vi "Read Data Type.vi"(8 "error in (no error)":errorcluster, 11 "Channel in":refnum<class "Channel.lvclass">) -> (0 "error out":errorcluster, 2 "Data Type":T1, 3 "Channel out":refnum<class "Channel.lvclass">)   [LabVIEW 2013, in "Channel.lvclass"]
uses:
  Channel.lvclass
  channel_dataType.ctl
  Channel.lvclass/Channel.ctl
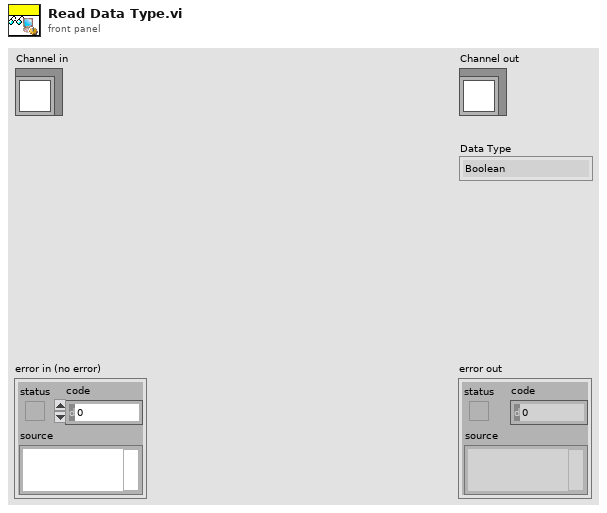
[diagram p1: front panel]
types:
  T1 = typedef "Channel.lvclass/channel_dataType.ctl" = enum16{"Boolean", "U8", "I8", "U16", "I16", "U32", "I32", "U64", "I64", "FXPI32", "FXPU32", "FXPI64", "FXPU64", "PWM"}
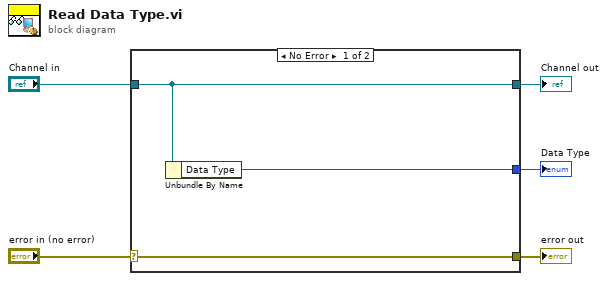
[diagram p0: block diagram]
diagram:
  n1 = case shown="No Error" "error in (no error)" {
    selector: "error in (no error)" -> [w8 w9]
    tunnel: [w8 w9] -> w4
    tunnel: [w7 w10] -> w2
    tunnel: "Channel in" -> [w7 w10]
    tunnel: [w6 _] -> w1
    frame No Error {
      n2 = Unbundle By Name(w7) -> ("Data Type"=w6:T1)
    }
    frame Error {
    }
  }
  "error out" <- w4
  "Channel out" <- w2
  "Data Type" <- w1
